vi "TestExec.Run Executable and Parse Results V2vi.vi"(6 "Reset":bool, 7 "Vars":variant, 8 "error in":errorcluster, 9 "Timeout(s)":dbl=500.0 caption="Time Out(s)" format="%.2f", 10 "Output Folder":path, 11 "Utility Config File":path) -> (0 "Error":errorcluster, 3 "RTN Data":T1 {"MeasData"."Status" items=["LOG", "PASS", "FAIL", "ERROR"]; "Attr"."Status" items=["LOG", "PASS", "FAIL", "ERROR"]; "Num"."Status" items=["LOG", "PASS", "FAIL", "ERROR"]})   [LabVIEW 2018]
uses:
  TestExec.Local Result Data.ctl
  Results/Result.Attribute.ctl
  Results/Result.Measurement and Attribute Item Status.ctl
  Results/Result.Numeric.ctl
  Results/Result.Limit Type.ctl
  Results/Result XML/TestResult.SW Item.ctl
  Reports/Report.Result FileDataObject.ctl
  Results/Result.Measurement Item.ctl
  Cmd Exe/CmdExe.Setup Params.ctl
  Cmd Exe/CmdExe.Output Error Check Setup.ctl
  <vilib>/KATE/Time/Time Utils.lvlib
panel:
  in  "Tab Control":enum32{"Execute", "Results"}(tab)
  out "Active":bool
  out "Sys Exec Commands":string
  out "Sys Exec STDOut":string
  out "Dur(s)":dbl caption="Duration(s)" format="%.3f"
  out "Rslt":u32(colorbox)=13816530 caption="Exe"
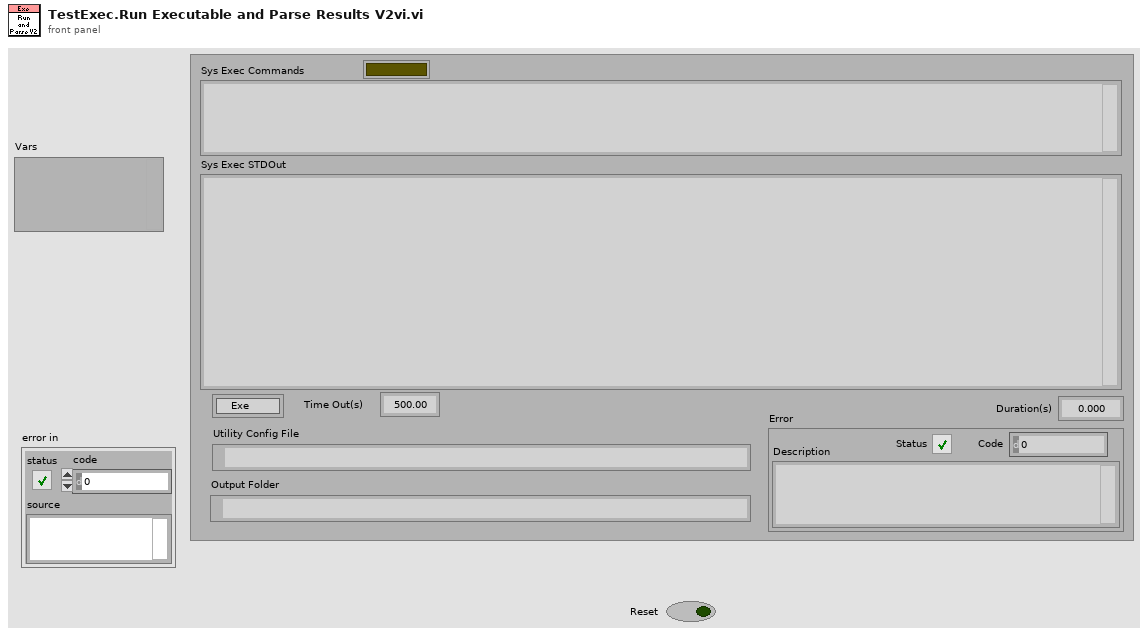
[diagram p1: front panel]
types:
  T1 = typedef "TestExec.Local Result Data.ctl" = cluster{"Attr":T2[], "Num":T4[], "UUT Props":string[][], "Vars":string[][], "SW Items":T6[], "Error":errorcluster, "Step":i32, "FileObjs":T7[], "MeasData":T8[]}
  T2 = typedef "Result.Attribute.ctl" = cluster{"Cnt":i32, "Step":string, "Category":string, "Name":string, "Value":string, "Status":T3, "Code":i32, "Desc":string, "Time":timestamp}
  T3 = typedef "Result.Measurement and Attribute Item Status.ctl" = i32
  T4 = typedef "Result.Numeric.ctl" = cluster{"Cnt":i32, "Step":string, "Category":string, "Name":string, "Value":dbl, "Units":string, "LimType":T5, "LL":dbl, "UL":dbl, "Status":T3, "Code":i32, "Desc":string, "Time":timestamp}
  T5 = typedef "Result.Limit Type.ctl" = enum16{"None", "EQ", "NE", "GT", "LT", "GE", "LE", "GTLT", "GELE", "GELT", "GTLE", "LTGT", "LEGE", "LEGT", "LTGE", "Contains", "NotContains"}
  T6 = typedef "TestResult.SW Item.ctl" = cluster{"Name":string, "PN":string, "Version":string, "Note":string}
  T7 = typedef "Report.Result FileDataObject.ctl" = cluster{"Cnt":i32, "Step":string, "Category":string, "Name":string, "Type":string, "File Name":string, "Time":string, "Path":path}
  T8 = typedef "Result.Measurement Item.ctl" = cluster{"Cnt":i32, "Step":string, "Category":string, "Name":string, "Value":string, "Units":string, "LimType":string, "LL":string, "UL":string, "Status":T3, "Code":i32, "Desc":string, "Time":timestamp}
  T9 = typedef "CmdExe.Setup Params.ctl" = cluster{"Timeout (s)":dbl, "Show Cmd Win":bool, "Error Check":T10, "Log_En":bool, "LogFileName":string, "LogDir":path}
  T10 = typedef "CmdExe.Output Error Check Setup.ctl" = cluster{"StdOut_Ck":bool, "StdOutErrMsgs":string[], "StdErr_Ck":bool, "RtnCode_Ck":bool, "RtnCodePASS":i32}
  T11 = cluster{"StdError":string, "RtnCode":i32, "Args":string, "Setup":T9, "StdOut":string, "ActionName":string, "Exe":path, "RTN Data":T1, "Prefix":string, "Code":i32, "OutputType":i32}
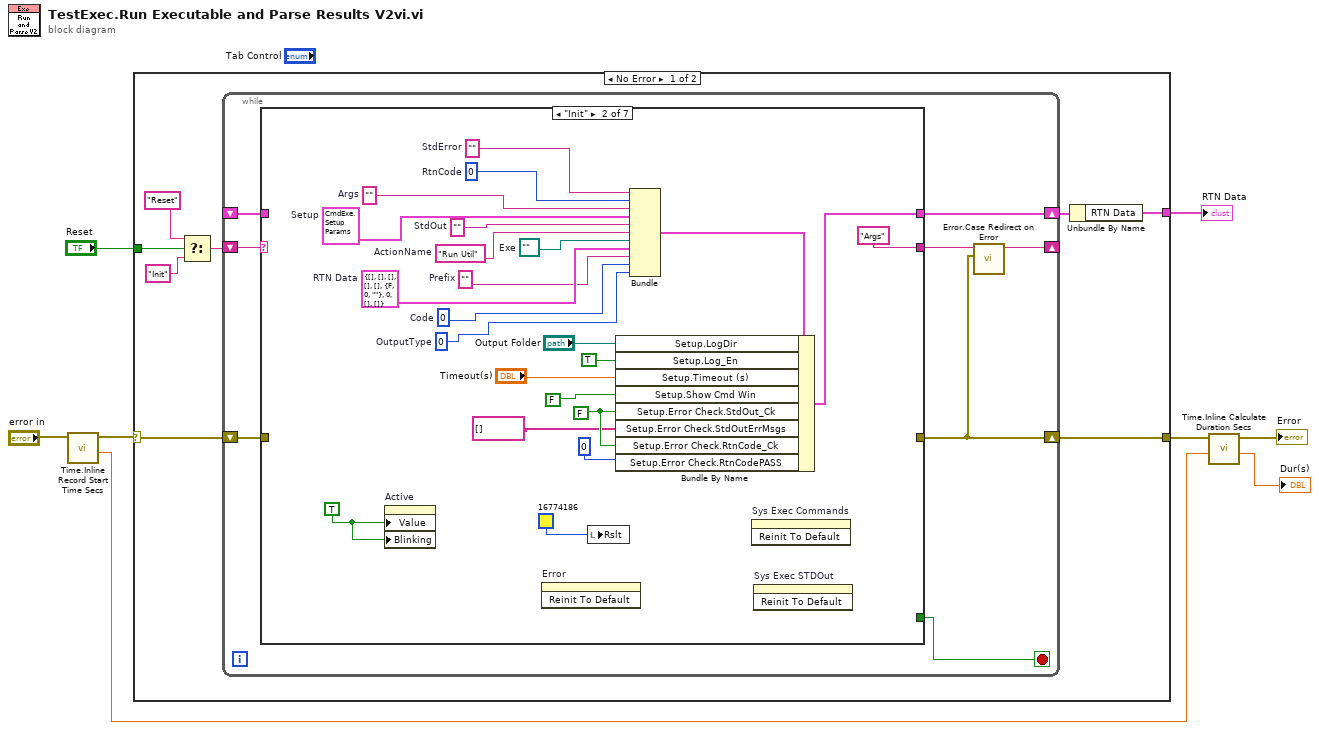
[diagram p0: block diagram]
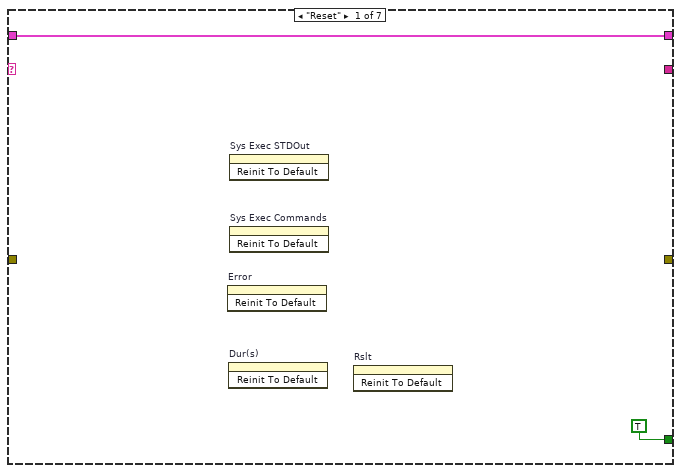
[diagram p2: hidden frame]
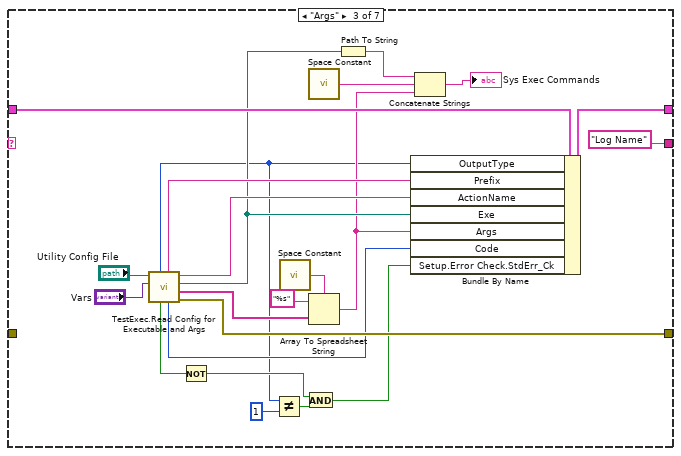
[diagram p3: hidden frame]
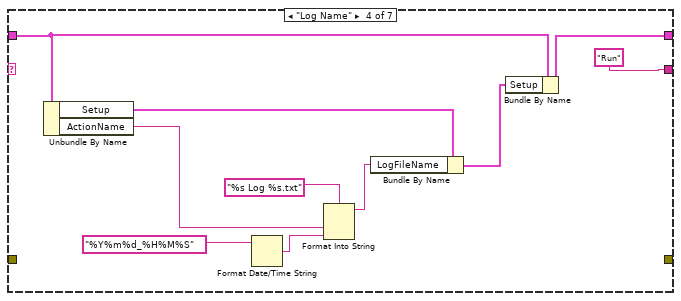
[diagram p4: hidden frame]
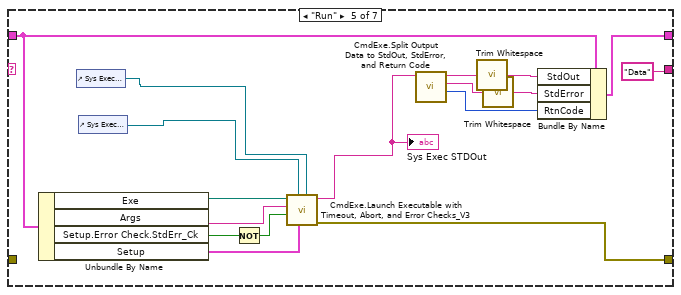
[diagram p5: hidden frame]
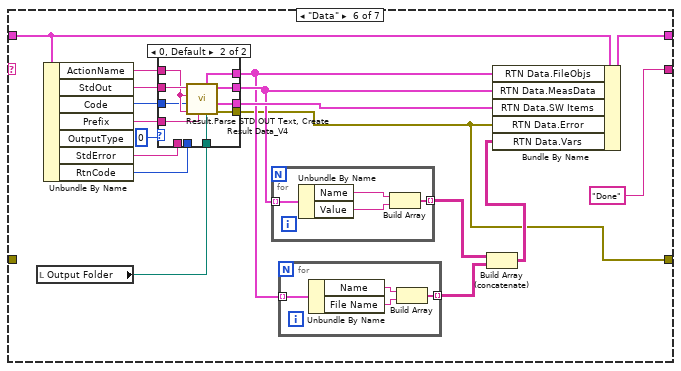
[diagram p6: hidden frame]
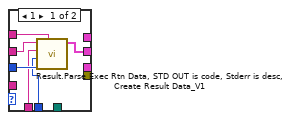
[diagram p7: hidden frame]
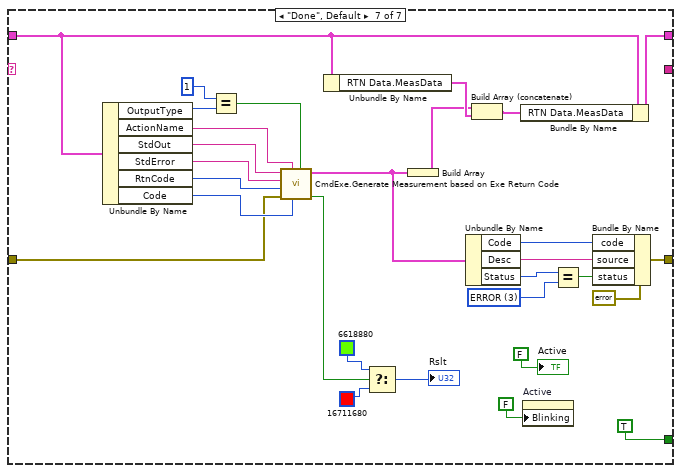
[diagram p8: hidden frame]
diagram:
  n1 = call <vilib>:"Time.Inline Record Start Time Secs.vi"("Error In Upper"="error in") -> ("Start(s)"=w2:dbl, "Error Out Upper"=w6:errorcluster)  [unwired: 8 in, 1 out]
  n2 = case shown="No Error" w6 {
    selector: w6 -> [w16 w170]
    tunnel: [w15 w170] -> w4
    tunnel: [w13 _] -> w8
    tunnel: "Reset" -> [w9 _]
    frame No Error {
      n3 = Select(t="Reset", s=w9, f="Init") -> (s? t:f=w11:string)
      n4 = while {
        shift-right: [w18] -> _
        shift-left: w11 -> [w24]
        shift-right: [w23] -> w14
        shift-left: _ -> [w22]
        shift-right: [w17] -> w15
        shift-left: w16 -> [w20]
        stop <- w21 stop-if-true
        n5 = case shown="\"Init\"" w24 {
          tunnel: [_ "Args" "Log Name" "Run" "Data" "Done" _] -> w19
          tunnel: [w26 w41 w72 w81 w90 w114 w160] -> w23
          tunnel: w22 -> [w26 _ w71 w80 w83 w113 w154]
          tunnel: [TRUE _ _ _ _ _ TRUE] -> w21
          tunnel: w20 -> [_ _ _ _ _ _ w153]
          tunnel: [_ _ w64 _ w89 w105 w145] -> w17
          frame "Reset" {
            n6 = invoke on="Error" class="Clust (strict)" method="Reinit To Default"() -> ()  [unwired: 3 in, 3 out]
            n7 = invoke on="Dur(s)" class="DigNum (strict)" method="Reinit To Default"() -> ()  [unwired: 3 in, 3 out]
            n8 = invoke on="Sys Exec STDOut" class="Str" method="Reinit To Default"() -> ()  [unwired: 3 in, 3 out]
            n9 = invoke on="Sys Exec Commands" class="Str" method="Reinit To Default"() -> ()  [unwired: 3 in, 3 out]
            n10 = invoke on="Rslt" class="ColBox" method="Reinit To Default"() -> ()  [unwired: 3 in, 3 out]
          }
          frame "Init" {
            w29 = 0  # RtnCode
            w28 = ""  # StdError
            w30 = 0  # OutputType
            w31 = 0  # Code
            w32 = ""  # Prefix
            w33 = T1 {"Attr"=[], "Num"=[], "UUT Props"=[], "Vars"=[], "SW Items"=[], "Error"={"status"=FALSE, "code"=0, "source"=""}, "Step"=0, "FileObjs"=[], "MeasData"=[]}  # RTN Data
            w34 = path ""  # Exe
            w35 = "Run Util"  # ActionName
            w38 = ""  # StdOut
            w42 = FALSE
            w47 = TRUE ("Value")
            w46 = T9 {"Timeout (s)"=60.0, "Show Cmd Win"=FALSE, "Error Check"={"StdOut_Ck"=FALSE, "StdOutErrMsgs"=["Error", "Unable to find device "], "StdErr_Ck"=FALSE, "RtnCode_Ck"=FALSE, "RtnCodePASS"=0}, "Log_En"=FALSE, "LogFileName"="", "LogDir"=path ""}  # Setup
            w49 = ""  # Args
            n11 = property on="Active" class="Bool (strict)"("Value"=w47, "Blinking"=w47) -> ()  [unwired: 2 in, 2 out]
            n12 = invoke on="Error" class="Clust (strict)" method="Reinit To Default"() -> ()  [unwired: 3 in, 3 out]
            n13 = local write "Rslt"(u32 16774186) -> ()
            n14 = Bundle("StdError"=w28, "RtnCode"=w29, "Args"=w49, "Setup"=w46, "StdOut"=w38, "ActionName"=w35, "Exe"=w34, "RTN Data"=w33, "Prefix"=w32, "Code"=w31, "OutputType"=w30) -> (w43:T11)  [unwired: 1 in]
            n15 = Bundle By Name(cluster=w43, "Setup.LogDir"="Output Folder", "Setup.Log_En"=TRUE, "Setup.Timeout (s)"="Timeout(s)", "Setup.Show Cmd Win"=FALSE, "Setup.Error Check.StdOut_Ck"=w42, "Setup.Error Check.StdOutErrMsgs"=string[] [], "Setup.Error Check.RtnCode_Ck"=w42, "Setup.Error Check.RtnCodePASS"=0 ("Error Check.RtnCodePASS")) -> (w41:T11)
            n16 = invoke on="Sys Exec Commands" class="Str" method="Reinit To Default"() -> ()  [unwired: 3 in, 3 out]
            n17 = invoke on="Sys Exec STDOut" class="Str" method="Reinit To Default"() -> ()  [unwired: 3 in, 3 out]
          }
          frame "Args" {
            n18 = call "TestExec.Read Config for Executable and Args.vi"("Vars"="Vars", "Config File"="Utility Config File") -> ("error out"=w64:errorcluster, "Args"=w66:string[], "Exe"=w58:path, "Action Name"=w63:string, "Error Code"=w62:i32, "Data Name Prefix"=w61:string, "IgnoreStdError"=w55:bool, "OutType"=w52:i32)  [unwired: 2 in]
            n19 = Not(x=w55) -> (.not. x?=w54:bool)
            n20 = Not Equal?(x=w52, y=1) -> (x != y?=w53:bool)
            n21 = call <vilib>:"Space Constant.vi"() -> ("String"=w67:string)
            n22 = And(x=w54, y=w53) -> (x .and. y?=w50:bool)
            n23 = call <vilib>:"Space Constant.vi"() -> ("String"=w56:string)
            n24 = Array To Spreadsheet String(delimiter (Tab)=w67, array=w66, 3:"%s" ("format string")) -> (spreadsheet string=w57:string)
            n25 = Path To String(path=w58) -> (string=w59:string)
            n26 = Bundle By Name(cluster=w71, "OutputType"=w52, "Prefix"=w61, "ActionName"=w63, "Exe"=w58, "Args"=w57, "Code"=w62, "Setup.Error Check.StdErr_Ck"=w50) -> (w72:T11)
            n27 = Concatenate Strings(w59, w56, w57) -> (→"Sys Exec Commands":string)
          }
          frame "Log Name" {
            n28 = Unbundle By Name(w80) -> ("Setup"=w78:T9, "ActionName"=w73:string)
            n29 = Format Date/Time String(time format string (%c)="%Y%m%d_%H%M%S") -> (date/time string=w74:string)  [unwired: 2 in]
            n30 = Format Into String(format string="%s Log %s.txt", w73, w74) -> (resulting string=w75:string)  [unwired: 2 in, 1 out]
            n31 = Bundle By Name(cluster=w78, "LogFileName"=w75) -> (w79:T9)
            n32 = Bundle By Name(cluster=w80, "Setup"=w79) -> (w81:T11)
          }
          frame "Run" {
            n33 = Unbundle By Name(w83) -> ("Exe"=w91:path, "Args"=w99:string, "Setup.Error Check.StdErr_Ck"=w88:bool, "Setup"=w98:T9)
            n34 = control-ref of="Sys Exec Commands"() -> (w97:refnum<vi>)
            n35 = control-ref of="Sys Exec STDOut"() -> (w96:refnum<vi>)
            n36 = Not(x=w88) -> (.not. x?=w87:bool)
            n37 = call "CmdExe.Launch Executable with Timeout, Abort, and Error Checks_V3.vi"("Cmd IN Ref"=w97, "Setup"=w98, "Output Ref"=w96, "Ignore StdErr"=w87, "Args"=w99, "Executable"=w91) -> ("error out"=w89:errorcluster, "Data Out"=w93:string)  [unwired: 2 in, 2 out]
            "Sys Exec STDOut" <- w93
            n38 = call "CmdExe.Split Output Data to StdOut, StdError, and Return Code.vi"("Output Data"=w93) -> ("Return Code"=w84:i32, "StdError"=w86:string, "StdOut"=w94:string)  [unwired: 7 in, 1 out]
            n39 = call <vilib>:"Trim Whitespace.vi"("string"=w94) -> ("trimmed string"=w92:string)  [unwired: 1 in]
            n40 = call <vilib>:"Trim Whitespace.vi"("string"=w86) -> ("trimmed string"=w85:string)  [unwired: 1 in]
            n41 = Bundle By Name(cluster=w83, "StdOut"=w92, "StdError"=w85, "RtnCode"=w84) -> (w90:T11)
          }
          frame "Data" {
            n42 = local read "Output Folder"() -> (w115:path)
            n43 = Unbundle By Name(w113) -> ("ActionName"=w110:string, "StdOut"=w117:string, "Code"=w104:i32, "Prefix"=w103:string, "StdError"=w102:string, "RtnCode"=w101:i32)  [unwired: 1 out]
            n44 = case shown="0, Default" 0 {
              tunnel: w117 -> [w122 w132]
              tunnel: [_ w131] -> w116
              tunnel: w115 -> [_ w130]
              tunnel: [w120 w129] -> w112
              tunnel: [_ w128] -> w111
              tunnel: w110 -> [w121 w127]
              tunnel: [_ w126] -> w105
              tunnel: w104 -> [w123 w125]
              tunnel: w103 -> [_ w124]
              tunnel: w102 -> [w119 _]
              tunnel: w101 -> [w118 _]
              frame 1 {
                n45 = call "Result.Parse Exec Rtn Data, STD OUT is code, Stderr is desc, Create Result Data_V1.vi"("Name"=w121, "BaseCode"=w123, "RtnCode"=w118, "StdErr"=w119, "StdOut"=w122) -> ("Meas"=w120:T8[])  [unwired: 6 in]
              }
              frame 0, Default {
                n46 = call "Result.Parse STD OUT Text, Create Result Data_V4.vi"("UUTDir"=w130, "Prefix"=w124, "Version Name"=w127, "Error Code"=w125, "Task Name"=w127, "StdOut"=w132) -> ("Error"=w126:errorcluster, "SW Ver"=w131:T6[], "Meas"=w129:T8[], "Data Files"=w128:T7[])  [unwired: 2 in]
              }
            }
            n47 = for {
              tunnel: w112 -> [w140] mode=indexing
              tunnel: [w137] -> w109 mode=indexing
              n48 = Unbundle By Name(w140) -> ("Name"=w139:string, "Value"=w138:string)
              n49 = Build Array(w139, w138) -> (w137:string[])
            }
            n50 = for {
              tunnel: w111 -> [w136] mode=indexing
              tunnel: [w134] -> w108 mode=indexing
              n51 = Unbundle By Name(w136) -> ("Name"=w135:string, "File Name"=w133:string)
              n52 = Build Array(w135, w133) -> (w134:string[])
            }
            n53 = Build Array (concatenate)(w109, w108) -> (w107:string[][])
            n54 = Bundle By Name(cluster=w113, "RTN Data.FileObjs"=w111, "RTN Data.MeasData"=w112, "RTN Data.SW Items"=w116, "RTN Data.Error"=w105, "RTN Data.Vars"=w107) -> (w114:T11)
          }
          frame "Done", Default {
            w147 = T3 3 items=["LOG", "PASS", "FAIL", "ERROR"] ("Status")
            n55 = Unbundle By Name(w154) -> ("OutputType"=w143:i32, "ActionName"=w159:string, "StdOut"=w158:string, "StdError"=w157:string, "RtnCode"=w156:i32, "Code"=w155:i32)
            n56 = Equal?(x=1, y=w143) -> (x = y?=w141:bool)
            n57 = call "CmdExe.Generate Measurement based on Exe Return Code.vi"("StdOut is Fail Code"=w141, "BaseCode"=w155, "Name"=w159, "Error"=w153, "RtnCode"=w156, "StdErr"=w157, "StdOut"=w158) -> ("Success"=w152:bool, "Meas"=w144:T8)  [unwired: 3 in]
            n58 = Unbundle By Name(w154) -> ("RTN Data.MeasData"=w163:T8[])
            n59 = Select(t=u32 6618880, s=w152, f=u32 16711680) -> (s? t:f=→"Rslt":u32)
            n60 = Build Array(w144) -> (w162:T8[])
            n61 = Unbundle By Name(w144) -> ("Code"=w149:i32, "Desc"=w150:string, "Status"=w148:T3)
            n62 = Build Array (concatenate)(w162, w163) -> (w164:T8[])
            n63 = Bundle By Name(cluster=w154, "RTN Data.MeasData"=w164) -> (w160:T11)
            n64 = property on="Active" class="Bool (strict)"("Blinking"=FALSE ("Value")) -> ()  [unwired: 2 in, 2 out]
            n65 = Equal?(x=w148, y=w147) -> (x = y?=w146:bool)
            n66 = Bundle By Name(cluster=errorcluster {"status"=FALSE, "code"=0, "source"=""} ("error constant"), "code"=w149, "source"=w150, "status"=w146) -> (w145:errorcluster)
            "Active" <- FALSE ("Active")
          }
        }
        n67 = call "Error.Case Redirect on Error.vi"("error in"=w17, "Next Case"=w19) -> ("Next Case Out"=w18:string)  [unwired: 9 in]
      }
      n68 = Unbundle By Name(w14) -> ("RTN Data"=w13:T1)
    }
    frame Error {
    }
  }
  "RTN Data" <- w8
  n69 = call <vilib>:"Time.Inline Calculate Duration Secs.vi"("Start(Sec)"=w2, "Error In Top"=w4) -> ("Duration(s)"=→"Dur(s)":dbl, "Error Out Top"=→"Error":errorcluster)  [unwired: 7 in, 1 out]
